vi "Write View Data.vi"(8 "error in (no error)":errorcluster, 10 "View Data":string[][](array[string]), 11 "List Box View Model in":refnum<class "Multicolumn List Box View Model.lvclass">) -> (0 "error out":errorcluster, 3 "List Box View Model out":refnum<class "Multicolumn List Box View Model.lvclass">)   [LabVIEW 2020, in "Multicolumn List Box View Model.lvclass"]
uses:
  Multicolumn List Box View Model.lvclass
  Multicolumn List Box View Model.lvclass/Multicolumn List Box View Model.ctl
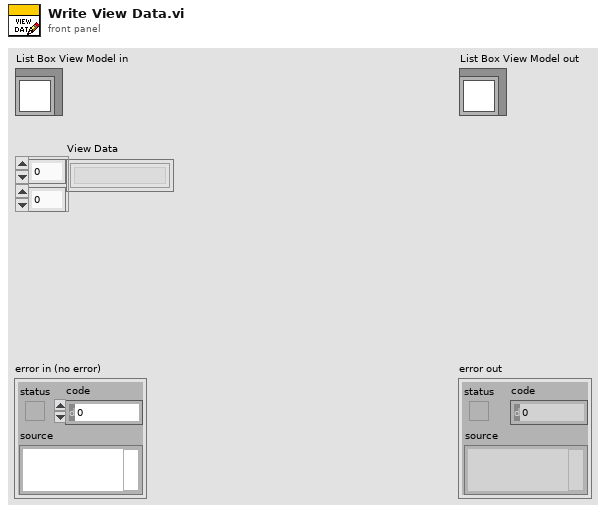
[diagram p1: front panel]
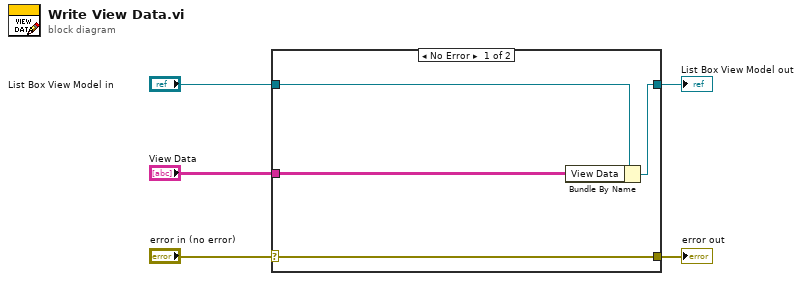
[diagram p0: block diagram]
diagram:
  n1 = case shown="No Error" "error in (no error)" {
    selector: "error in (no error)" -> [w9 w10]
    tunnel: [w9 w10] -> w4
    tunnel: [w7 w11] -> w2
    tunnel: "List Box View Model in" -> [w8 w11]
    tunnel: "View Data" -> [w6 _]
    frame No Error {
      n2 = Bundle By Name(cluster=w8, "View Data"=w6) -> (w7:refnum<class "Multicolumn List Box View Model.lvclass">)
    }
    frame Error {
    }
  }
  "error out" <- w4
  "List Box View Model out" <- w2
